vi "Initialize Front Panel.vi"(8 "error in (no error)":errorcluster, 11 "SimpleChart in":refnum<class "SimpleChart.lvclass">) -> (0 "error out":errorcluster, 3 "SimpleChart out":refnum<class "SimpleChart.lvclass">)   [LabVIEW 2017, in "MVAExamples.lvlib" / "SimpleChart.lvclass"]
doc: "<License>\nCopyright © 2017 Composed Systems, LLC | All rights reserved\nwww.composed.io\n\nAuthor: Ethan Stern <ethan.stern@composed.io>\n\nThis software is provided \"AS IS\" WITHOUT WARRANTIES, either express or implied, AND IS FOR EDUCATIONAL PURPOSES ONLY.\n</License>"
uses:
  SimpleChart.lvclass
  SimpleChart.lvclass/SimpleChart.ctl
  Source/Framework/IViewable/IViewable/IViewable.lvclass
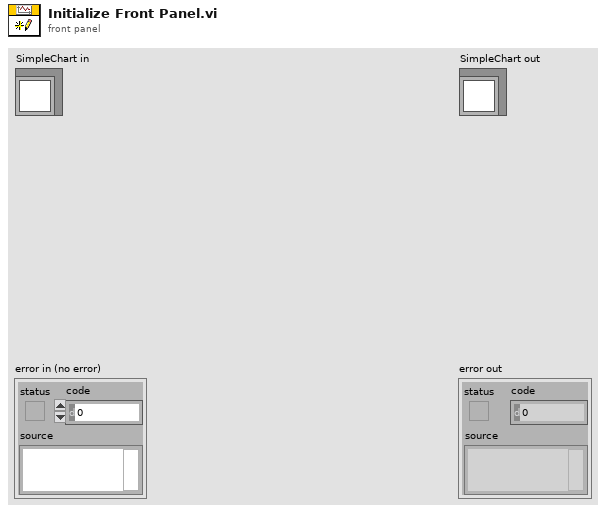
[diagram p1: front panel]
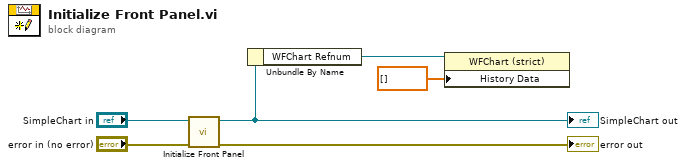
[diagram p0: block diagram]
diagram:
  n1 = call-parent "Initialize Front Panel.vi"("error in (no error)"="error in (no error)", "IViewable in"="SimpleChart in") -> ("error out"=→"error out":errorcluster, "IViewable out"=w3:refnum<class "SimpleChart.lvclass">)  [unwired: 8 in]
  "SimpleChart out" <- w3
  n2 = Unbundle By Name(w3) -> ("WFChart Refnum"=w2:refnum<vi>)
  n3 = property class="WFChart (strict)"(reference=w2, "History Data"=dbl[] []) -> ()  [unwired: 1 in, 2 out]
